vi "Do.vi"(8 "error in (no error)":errorcluster, 10 "Actor in":refnum<class "Actor.lvclass">, 11 "Update a Dev Requested by UI Msg":refnum<class "Update a Dev Requested by UI Msg.lvclass">) -> (0 "error out":errorcluster, 2 "Actor out":refnum<class "Actor.lvclass">)   [LabVIEW 2016, in "Controller Actor.lvlib" / "Update a Dev Requested by UI Msg.lvclass"]
uses:
  <userlib>/Common Components/Controller/Messages/Update a Dev Requested by UI Msg/Update a Dev Requested by UI Msg.lvclass
  <vilib>/ActorFramework/Actor/Actor.lvclass
  <userlib>/Common Components/Controller/Controller.lvclass
  C:/Program Files (x86)/National Instruments/LabVIEW 2016/vi.lib/ActorFramework/Actor/Actor.lvclass
  <userlib>/Common Components/Controller/Messages/Update a Dev Requested by UI Msg/Update a Dev Requested by UI Msg.lvclass/Update a Dev Requested by UI Msg.ctl
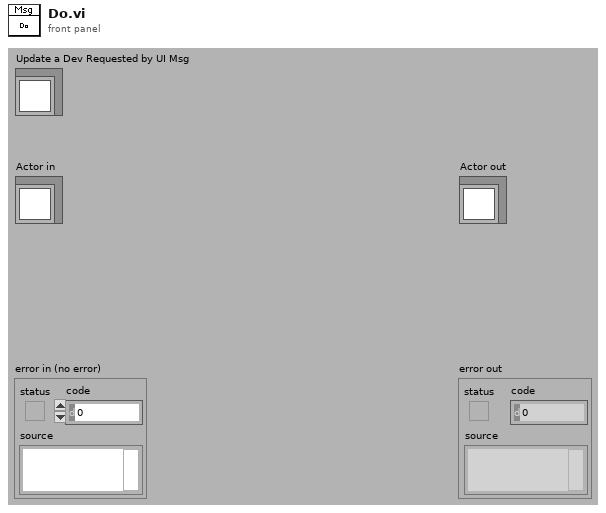
[diagram p1: front panel]
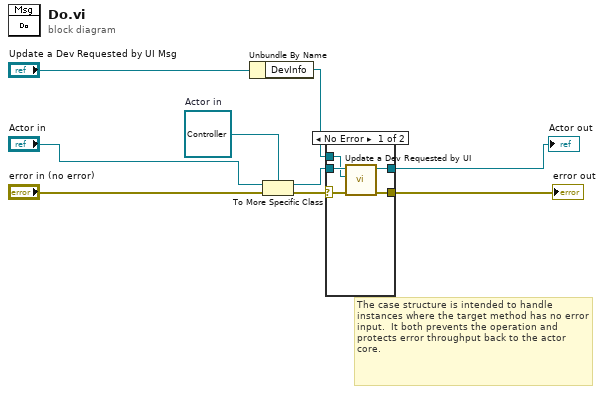
[diagram p0: block diagram]
diagram:
  w5 = refnum<class "Controller.lvclass"> refnum  # Actor in
  # "The case structure is intended to handle instances where the target method has no error input.  It both prevents the operation and protects error throughput back to the actor core."
  n1 = Unbundle By Name("Update a Dev Requested by UI Msg") -> ("DevInfo"=w1:refnum<class "DevInfo.lvclass">)
  n2 = To More Specific Class(target class=w5, reference="Actor in", error in="error in (no error)") -> (specific class reference=w8:refnum<class "Controller.lvclass">, error out=w4:errorcluster)
  n3 = case shown="No Error" w4 {
    selector: w4 -> [w11 w16]
    tunnel: w8 -> [w14 w15]
    tunnel: [w13 w16] -> w3
    tunnel: [w12 w15] -> w2
    tunnel: w1 -> [w10 _]
    frame No Error {
      n4 = call-dynamic "Update a Dev Requested by UI.vi"("error in (no error)"=w11, "DevInfo"=w10, "Controller in"=w14) -> ("error out"=w13:errorcluster, "Controller out"=w12:refnum<class "Controller.lvclass">)  [unwired: 7 in]
    }
    frame Error {
    }
  }
  "error out" <- w3
  "Actor out" <- w2
